vi "RS - Reset the controller.vi"(6 "error in":errorcluster, 9 "Address / Port":i16=1 min=1 max=31 step=1) -> (0 "error out":errorcluster, 3 "Address / Port out":i16)   [LabVIEW 2014]
doc: "Resets the ESP300 controller. The reset operation takes up to 20 seconds."
panel:
  # "RESETTING THE ESP300 CONTROLLER"
  # "This operation can last up to 20 seconds"
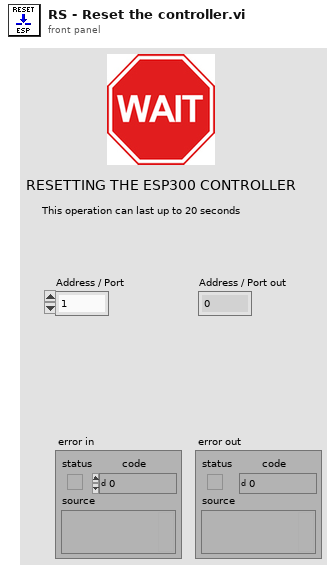
[diagram p1: front panel]
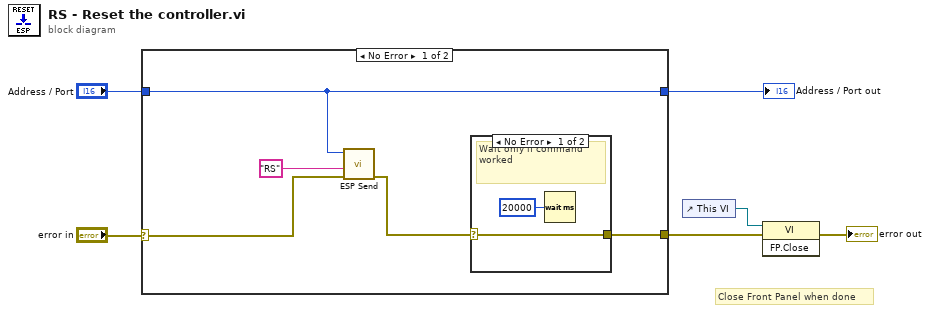
[diagram p0: block diagram]
diagram:
  # "Close Front Panel when done"
  n1 = case shown="No Error" "error in" {
    selector: "error in" -> [w10 w16]
    tunnel: "Address / Port" -> [w9 w15]
    tunnel: [w7 w16] -> w2
    tunnel: [w9 w15] -> w4
    frame No Error {
      n2 = call "ESP Send.vi"("error in"=w10, "Command String"="RS" ("Substring"), "Address / Port"=w9) -> ("error out"=w8:errorcluster)  [unwired: 3 in, 1 out]
      n3 = case shown="No Error" w8 {
        selector: w8 -> [w12 w14]
        tunnel: [w12 w14] -> w7
        frame No Error {
          # "Wait only if command worked"
          n4 = Wait (ms)(milliseconds to wait=u32 20000) -> ()  [unwired: 1 out]
        }
        frame Error {
          # "Pass error at output"
        }
      }
    }
    frame Error {
    }
  }
  "Address / Port out" <- w4
  n5 = control-ref of="This VI"() -> (w3:refnum<vi>)
  n6 = invoke class="VI" method="FP.Close"(reference=w3, error in=w2) -> (error out=→"error out":errorcluster)  [unwired: 1 in, 2 out]
